vi "getAnalogOutput.vi"(8 "error in (no error)":errorcluster, 11 "AoDeviceData.lvclass in":refnum<class "AoDeviceData.lvclass">) -> (0 "error out":errorcluster, 2 "aOChannel":refnum<class "AnalogOutput.lvclass">, 3 "AoDeviceData.lvclass out":refnum<class "AoDeviceData.lvclass">)   [LabVIEW 2009, in "DataMappers.lvlib" / "AoDeviceData.lvclass"]
uses:
  AoDeviceData.lvclass
  Hal/Channels/VoltOutput/AnalogOutput.lvclass
  AoDeviceData.lvclass/AoDeviceData.ctl
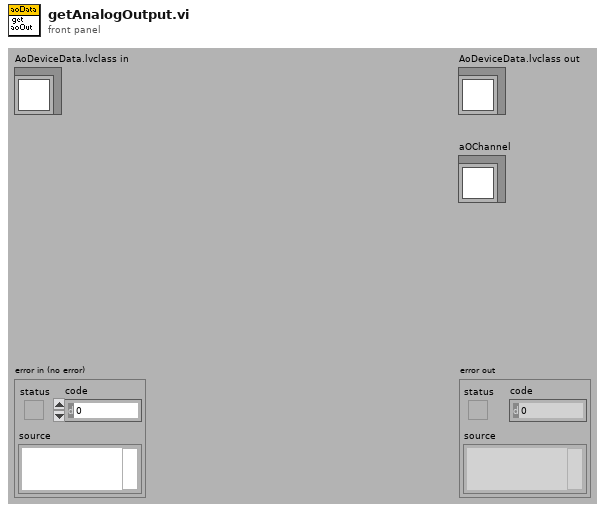
[diagram p1: front panel]
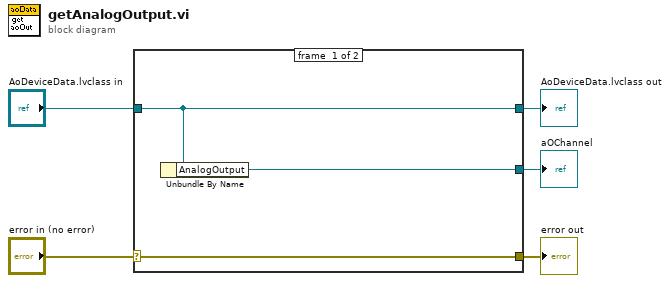
[diagram p0: block diagram]
diagram:
  n1 = case shown="No Error" "error in (no error)" {
    selector: "error in (no error)" -> [w8 w9]
    tunnel: [w8 w9] -> w4
    tunnel: [w7 w10] -> w2
    tunnel: "AoDeviceData.lvclass in" -> [w7 w10]
    tunnel: [w6 _] -> w1
    frame #0 {
      n2 = Unbundle By Name(w7) -> ("AnalogOutput"=w6:refnum<class "AnalogOutput.lvclass">)
    }
    frame #1 {
    }
  }
  "error out" <- w4
  "AoDeviceData.lvclass out" <- w2
  "aOChannel" <- w1
